vi "CLSUIP_UserScripting.vi"(8 "error in":errorcluster, 10 "VI Refnum in":refnum<vi>, 11 "VIRetooler":refnum<class "OverrideRetooler.lvclass">) -> (0 "error out":errorcluster, 3 "VIRetooler out":refnum<class "OverrideRetooler.lvclass">)   [LabVIEW 2021, in "MemberVICreation.lvlib" / "OverrideRetooler.lvclass"]
doc: "This VI does nothing. It provides an opportunity for users to add scripting code of their own to modify the retooling process even if they do not have the password to the VIs in the retooling process. Each overriding class should call out to an empty subVI, one that is not a member of the class, that users can edit to put in their own scripting behavior."
uses:
  <resource>/Framework/Providers/LVClassLibrary/NewAccessors/OverrideRetooler/OverrideRetooler.lvclass
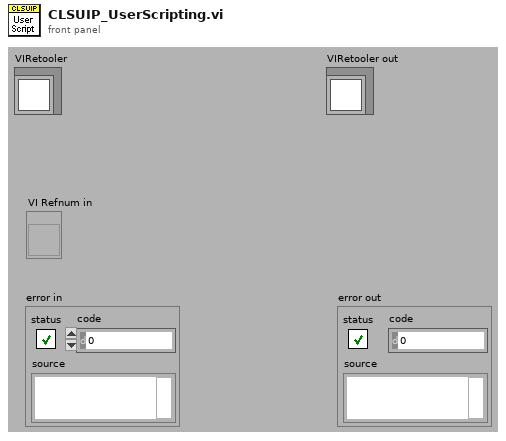
[diagram p1: front panel]
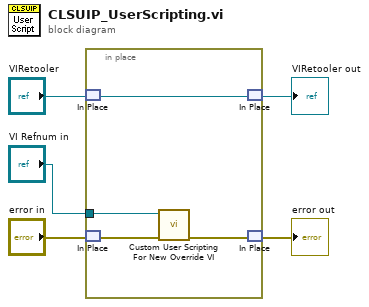
[diagram p0: block diagram]
diagram:
  n1 = in-place {
    in-place-border: "VI Refnum in" -> [w6]
    n2 = in-place-match #1("VIRetooler") -> (w9:refnum<class "OverrideRetooler.lvclass">)
    n3 = in-place-match #2("error in") -> (w7:errorcluster)
    n4 = call <resource>:"Custom User Scripting For New Override VI.vi"("error in"=w7, "VI Refnum in"=w6) -> ("error out"=w8:errorcluster)  [unwired: 9 in]
    n5 = in-place-match #1(w9) -> (→"VIRetooler out":refnum<class "OverrideRetooler.lvclass">)
    n6 = in-place-match #2(w8) -> (→"error out":errorcluster)
  }
